vi "Set Display names.vi"() -> ()   [LabVIEW 2020]
uses:
  <vilib>/Utility/config.llb/Read Key (String).vi
  <vilib>/Utility/config.llb/NI_LVConfig.lvlib
  <vilib>/LabVIEW Icon API/Set Text Icon/Text-Based VI Icon.lvlib
panel:
  out "section exists?":bool
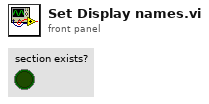
[diagram p1: front panel]
types:
  T1 = typedef "NI_LVConfig.lvlib/Config Data RefNum.ctl" = refnum<k1>
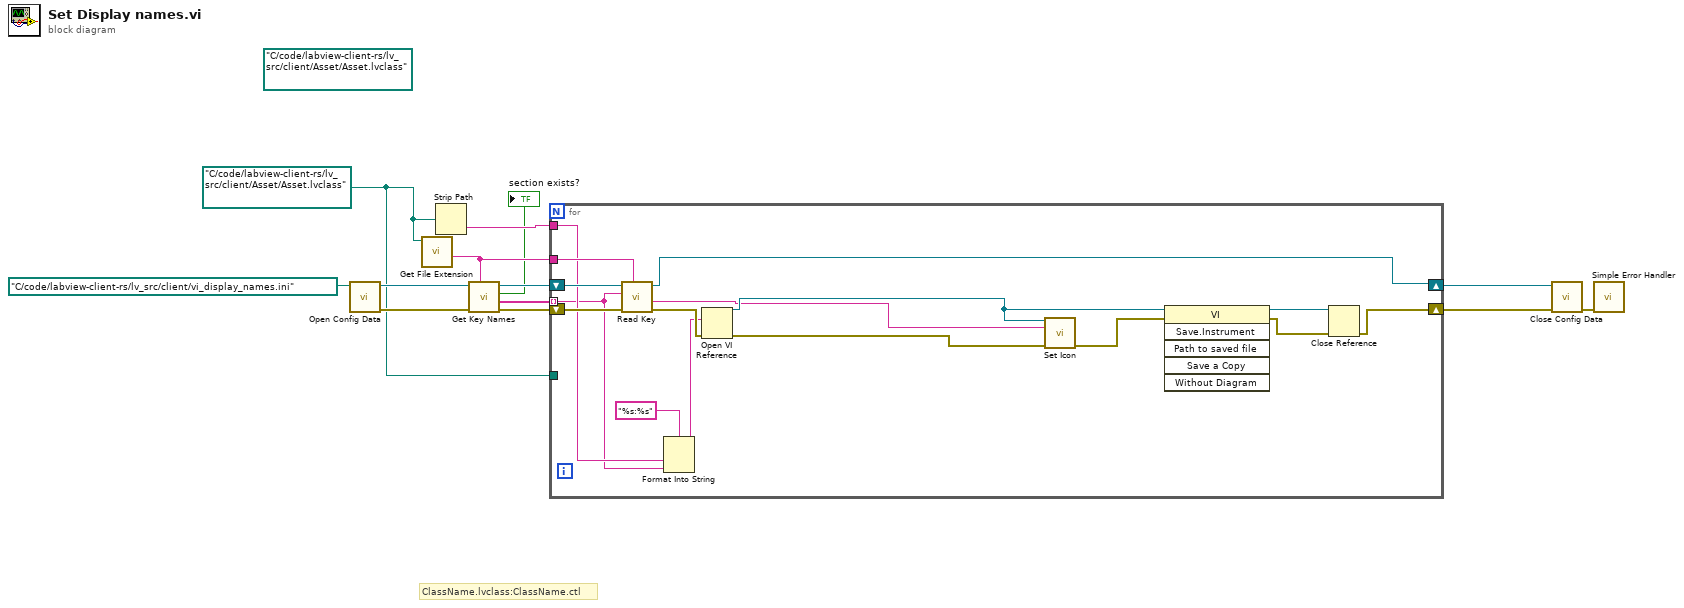
[diagram p0: block diagram]
diagram:
  (unwired) path "C:/code/labview-client-rs/lv_src/client/Asset/Asset.lvclass" ("Path")
  w1 = path "C:/code/labview-client-rs/lv_src/client/Asset/Asset.lvclass" ("Path")
  # "ClassName.lvclass:ClassName.ctl"
  n1 = call <vilib>:"Open Config Data.vi"("configuration file path"=path "C:/code/labview-client-rs/lv_src/client/vi_display_names.ini") -> ("error out"=w11:errorcluster, "refnum"=w2:T1)  [unwired: 8 in, 1 out]
  n2 = call <vilib>:"Get File Extension.vi"("file"=w1) -> ("filename without extension"=w8:string)  [unwired: 6 in, 4 out]
  n3 = Strip Path(path=w1) -> (name=w6:string)  [unwired: 1 out]
  n4 = call <vilib>:"Get Key Names.vi"("section"=w8, "error in (no error)"=w11, "refnum"=w2) -> ("error out"=w7:errorcluster, "key names"=w10:string[], "section exists?"=→"section exists?":bool, "refnum out"=w9:T1)  [unwired: 5 in]
  n5 = for {
    tunnel: w10 -> [w15] mode=indexing
    tunnel: w8 -> [w27]
    tunnel: w6 -> [w20]
    shift-right: [w25] -> w5
    shift-left: w9 -> [w26]
    shift-right: [w23] -> w4
    shift-left: w7 -> [w24]
    tunnel: w1 -> [_]
    n6 = call-poly <vilib>:"Read Key.vi"("section"=w27, "error in (no error)"=w24, "key"=w15, "refnum"=w26) -> ("error out"=w22:errorcluster, "value"=w14:string, "refnum out"=w25:T1)  [unwired: 4 in, 1 out]
    n7 = Format Into String(format string="%s:%s", w20, w15) -> (resulting string=w19:string)  [unwired: 2 in, 1 out]
    n8 = Open VI Reference(vi path=w19, error in (no error)=w22) -> (vi reference=w16:refnum<vi>, error out=w17:errorcluster)  [unwired: 4 in]
    n9 = call <vilib>:"Set Icon.vi"("VI"=w16, "user-supplied text (\"\" - use VI file name)"=w14, "error in"=w17) -> ("error out"=w18:errorcluster)  [unwired: 11 in, 1 out]
    n10 = invoke class="VI" method="Save.Instrument"(reference=w16, error in=w18) -> (reference out=w28:refnum<vi>, error out=w29:errorcluster)  [unwired: 4 in, 4 out]
    n11 = Close Reference(reference=w28, error in (no error)=w29) -> (error out=w23:errorcluster)
  }
  n12 = call <vilib>:"Close Config Data.vi"("error in (no error)"=w4, "refnum"=w5) -> ("error out"=w13:errorcluster)  [unwired: 8 in, 1 out]
  n13 = call <vilib>:"Simple Error Handler.vi"("error in (no error)"=w13) -> ()  [unwired: 4 in, 5 out]
